vi "OAT Timebase Plot Indicator.vi"() -> ()   [LabVIEW 2017]
doc: "Uses the Timebase Plot to display the amplitude of even angle signal or magnitude of a certain order as a function of time on a customized XY graph."
uses:
  <vilib>/addons/Sound and Vibration/Order Analysis/Backward Compatibility/SubVIs/oa_Timebase Plot Control.ctl
  <vilib>/addons/Sound and Vibration/Order Analysis/Backward Compatibility/OAT Timebase Plot (Unfiltered).vi
panel:
  out "Y axis":T1
  out "X axis":T1
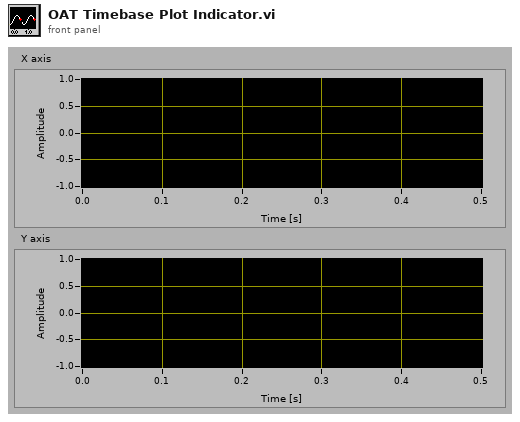
[diagram p1: front panel]
types:
  T1 = typedef "oa_Timebase Plot Control.ctl" = cluster{"X":dbl[], "Y":dbl[]}[]
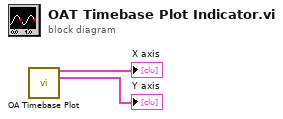
[diagram p0: block diagram]
diagram:
  n1 = call-poly <vilib>:"OA Timebase Plot.vi"() -> ("x-axis"=→"X axis":T1, "y-axis"=→"Y axis":T1)  [unwired: 13 in, 1 out]
